vi "As PropertyObject.vi"(8 "error in (no error)":errorcluster, 11 "Report in":refnum<class "Report.lvclass">) -> (0 "error out":errorcluster, 2 "PropertyObject":refnum<k7>, 3 "Report out":refnum<class "Report.lvclass">)   [LabVIEW 2020, in "TSnax.lvlib" / "Report.lvclass"]
uses:
  Report.lvclass
  Report.lvclass/Report.ctl
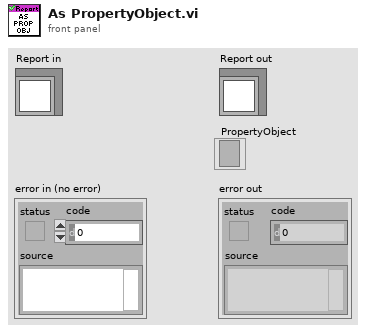
[diagram p1: front panel]
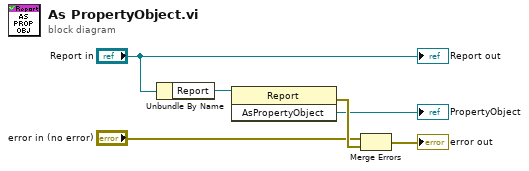
[diagram p0: block diagram]
diagram:
  n1 = Unbundle By Name("Report in") -> ("Report"=w3:refnum<k7>)
  n2 = invoke class="Report" method="AsPropertyObject"(reference=w3) -> (error out=w6:errorcluster, "AsPropertyObject"=→"PropertyObject":refnum<k7>)  [unwired: 2 in, 1 out]
  n3 = Merge Errors("error in (no error)", w6) -> (→"error out":errorcluster)
  "Report out" <- "Report in"
